vi "Configure NF Frequency.vi"(0 "VISA resource name":refnum<visa-resource-name>, 1 "Fixed Frequency Value (1.505 GHz)":dbl=1505000000.0 format="%^#_6g", 5 "Frequency Mode (0: Sweep)":u16(ring) items=["Sweep", "Fixed", "List"], 7 "Start Frequency (10 MHz)":dbl=10000000.0 format="%^#_6g", 9 "Stop Frequency (3 GHz)":dbl=3000000000.0 format="%^#_6g", 11 "error in (no error)":errorcluster, 12 "Frequency List (Hz)":dbl[](array[numeric]) format="%^#_6g") -> (4 "VISA resource name out":refnum<visa-resource-name>, 15 "error out":errorcluster)   [LabVIEW 2014, in "Agilent ESA PSA Series.lvlib"]
doc: "Selects the frequency mode and configures the selected mode for the Noise Figure personality.\n\n<B>Note:</B> \n\nThis VI is only valid in Noise Figure personality. Use <B>Switch Personality</B> VI to switch to Noise Figure before calling this VI."
uses:
  Agilent ESA PSA Series.lvlib
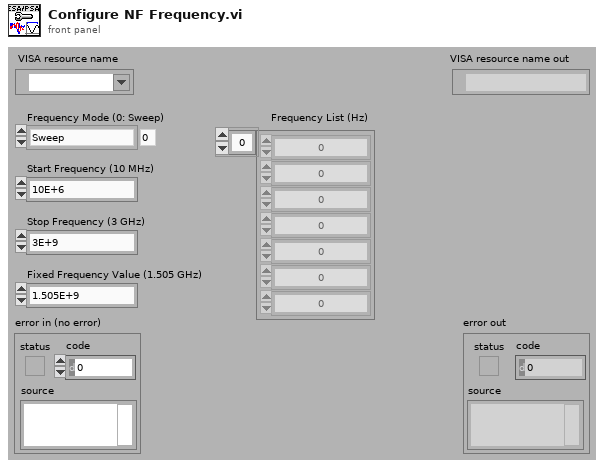
[diagram p1: front panel]
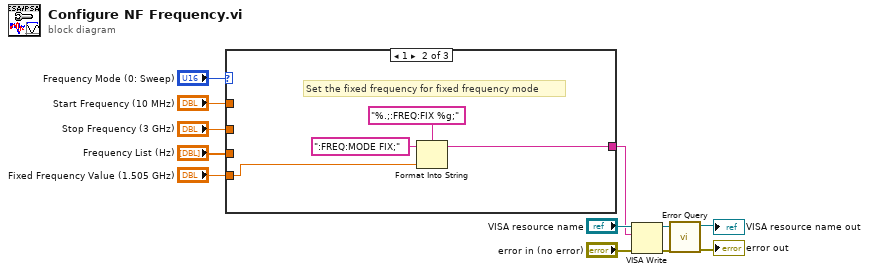
[diagram p0: block diagram]
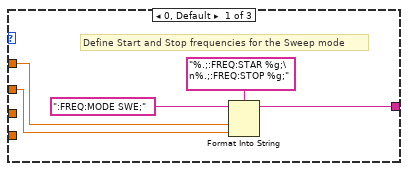
[diagram p2: hidden frame]
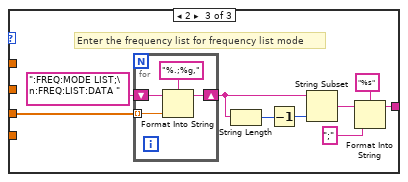
[diagram p3: hidden frame]
diagram:
  n1 = case shown="1" "Frequency Mode (0: Sweep)" {
    tunnel: "Frequency List (Hz)" -> [_ _ w29]
    tunnel: [w14 w21 w22] -> w1
    tunnel: "Start Frequency (10 MHz)" -> [w17 _ _]
    tunnel: "Stop Frequency (3 GHz)" -> [w16 _ _]
    tunnel: "Fixed Frequency Value (1.505 GHz)" -> [_ w19 _]
    frame 0, Default {
      # "Define Start and Stop frequencies for the Sweep mode"
      n2 = Format Into String(format string="%.;:FREQ:STAR %g;\n%.;:FREQ:STOP %g;", initial string=":FREQ:MODE SWE;", w17, w16) -> (resulting string=w14:string)  [unwired: 1 in, 1 out]
    }
    frame 1 {
      # "Set the fixed frequency for fixed frequency mode"
      n3 = Format Into String(format string="%.;:FREQ:FIX %g;", initial string=":FREQ:MODE FIX;", w19) -> (resulting string=w21:string)  [unwired: 1 in, 1 out]
    }
    frame 2 {
      # "Enter the frequency list for frequency list mode"
      n4 = for {
        shift-right: [w33] -> w25
        shift-left: ":FREQ:MODE LIST;\n:FREQ:LIST:DATA " -> [w34]
        tunnel: w29 -> [w31] mode=indexing
        n5 = Format Into String(format string="%.;%g,", initial string=w34, w31) -> (resulting string=w33:string)  [unwired: 1 in, 1 out]
      }
      n6 = String Length(string=w25) -> (length=w27:i32)
      n7 = Decrement(x=w27) -> (x-1=w28:i32)
      n8 = String Subset(string=w25, length (rest)=w28) -> (substring=w26:string)  [unwired: 1 in]
      n9 = Format Into String(format string="%s", initial string=w26, ";" ("input 1")) -> (resulting string=w22:string)  [unwired: 1 in, 1 out]
    }
  }
  n10 = VISA Write(VISA resource name="VISA resource name", write buffer=w1, error in (no error)="error in (no error)") -> (VISA resource name out=w7:refnum<visa-resource-name>, error out=w9:errorcluster)  [unwired: 1 out]
  n11 = call "Error Query.vi"("error in (no error)"=w9, "VISA resource name"=w7) -> ("error out"=→"error out":errorcluster, "VISA resource name out"=→"VISA resource name out":refnum<visa-resource-name>)  [unwired: 6 in, 2 out]
